vi "Example-DigitalOutSimple.vi"() -> ()   [LabVIEW 2018]
panel:
  in  "trigsrc":T1(ring)
  in  "trigcond":enum16{"Raising", "Falling", "Either"}(ring)
  out "Frequency(Hz)":i32=9600
  in  "divinit":u32
  in  "div":u32=1
  in  "type":enum16{"Pluse", "Custom", "Random"}(ring)
  in  "counter_h":u32=1
  in  "counter_l":u32=1
  in  "initlevel":i32
  in  "counter":u32
  in  "idle":i32
  in  "chs":u32=8 format="%.0x"
  in  "output":bool=TRUE
  out "returns":i32
  out "error out":errorcluster caption="错误输出"
  in  "error in (no error)":errorcluster caption="错误输入（无错误）"
  out "ftHandle out":u64
  in  "设备索引":i32
  # "单通道4为例"
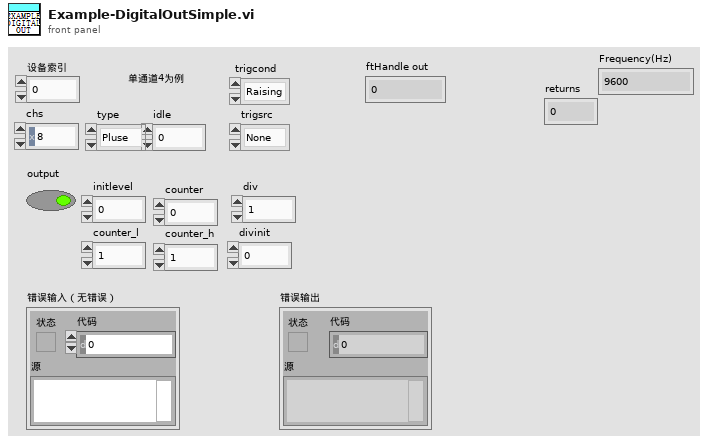
[diagram p1: front panel]
types:
  T1 = enum16{"None", "DetectorAnalogInCH1", "DetectorAnalogInCH2", "AnalogOut1", "AnalogOut2", "DetectorDigitalIn", "DigitalOut", "Manule", "External 1", "External 2", "DigitalIn"}
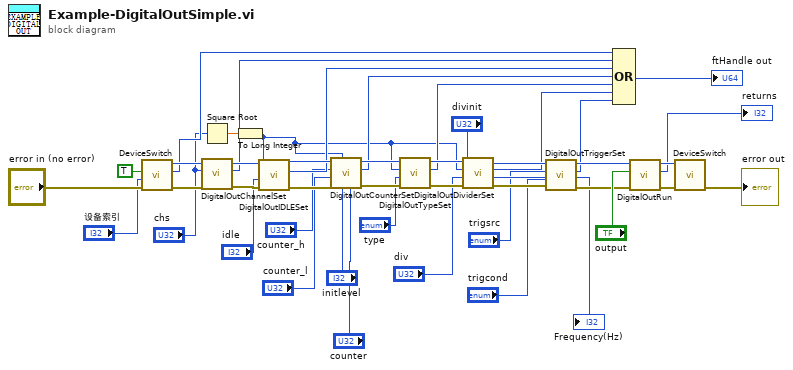
[diagram p0: block diagram]
diagram:
  n1 = call "DeviceSwitch.vi"("error in (no error)"="error in (no error)", "Device Index"="设备索引", "Open"=TRUE) -> ("error out"=w36:errorcluster, "function return"=w15:i32, "handle out"=w35:u64)  [unwired: 4 in, 2 out]
  n2 = Square Root(x="chs") -> (sqrt(x)=w13:dbl)
  n3 = call "DigitalOutChannelSet.vi"("error in (no error)"=w36, "chs"="chs", "handle"=w35) -> ("error out"=w34:errorcluster, "function return"=w17:i32, "handle out"=w23:u64)  [unwired: 6 in]
  n4 = To Long Integer(number=w13) -> (32bit integer=w12:i32)
  n5 = call "DigitalOutIDLESet.vi"("error in (no error)"=w34, "idle"="idle", "ch"=w12, "handle"=w23) -> ("error out"=w33:errorcluster, "function return"=w18:i32, "handle out"=w24:u64)  [unwired: 5 in]
  n6 = call "DigitalOutCounterSet.vi"(4:"counter_l"="counter", "initlevel"="initlevel", "ch"=w12, "error in (no error)"=w33, 9:"counter_l"="counter_l", "counter_h"="counter_h", "handle"=w24) -> ("error out"=w32:errorcluster, "function return"=w19:i32, "handle out"=w25:u64)  [unwired: 2 in]
  n7 = call "DigitalOutTypeSet.vi"("error in (no error)"=w32, "type"="type", "ch"=w12, "handle"=w25) -> ("error out"=w31:errorcluster, "function return"=w20:i32, "handle out"=w26:u64)  [unwired: 5 in]
  n8 = call "DigitalOutDividerSet.vi"("divinit"="divinit", "error in (no error)"=w31, "div"="div", "ch"=w12, "handle"=w26) -> ("error out"=w30:errorcluster, "Frequency(Hz)"=→"Frequency(Hz)":i32, "function return"=w21:i32, "handle out"=w27:u64)  [unwired: 3 in]
  n9 = call "DigitalOutTriggerSet.vi"("error in (no error)"=w30, "trigcond"="trigcond", "trigsrc"="trigsrc", "handle"=w27) -> ("error out"=w29:errorcluster, "function return"=w22:i32, "handle out"=w28:u64)  [unwired: 5 in]
  n10 = Compound Arithmetic op=OR ("复合运算")(w15, w17, w18, w19, w20, w21, w22) -> (→"ftHandle out":i32)
  n11 = call "DigitalOutRun.vi"("error in (no error)"=w29, "RUN"="output", "handle"=w28) -> ("error out"=w39:errorcluster, "function return"=→"returns":i32, "handle out"=w38:u64)  [unwired: 6 in]
  n12 = call "DeviceSwitch.vi"("error in (no error)"=w39, "handle"=w38) -> ("error out"=→"error out":errorcluster)  [unwired: 5 in, 4 out]
